vi "Day05-1.vi"() -> ()   [LabVIEW 2021]
panel:
  out "points with at least two lines overlap":i32
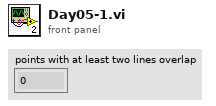
[diagram p1: front panel]
types:
  T1 = cluster{"[0]":i32, "[1]":i32, "[2]":i32, "[3]":i32, "[4]":i32, "[5]":i32, "[6]":i32, "[7]":i32, "[8]":i32}
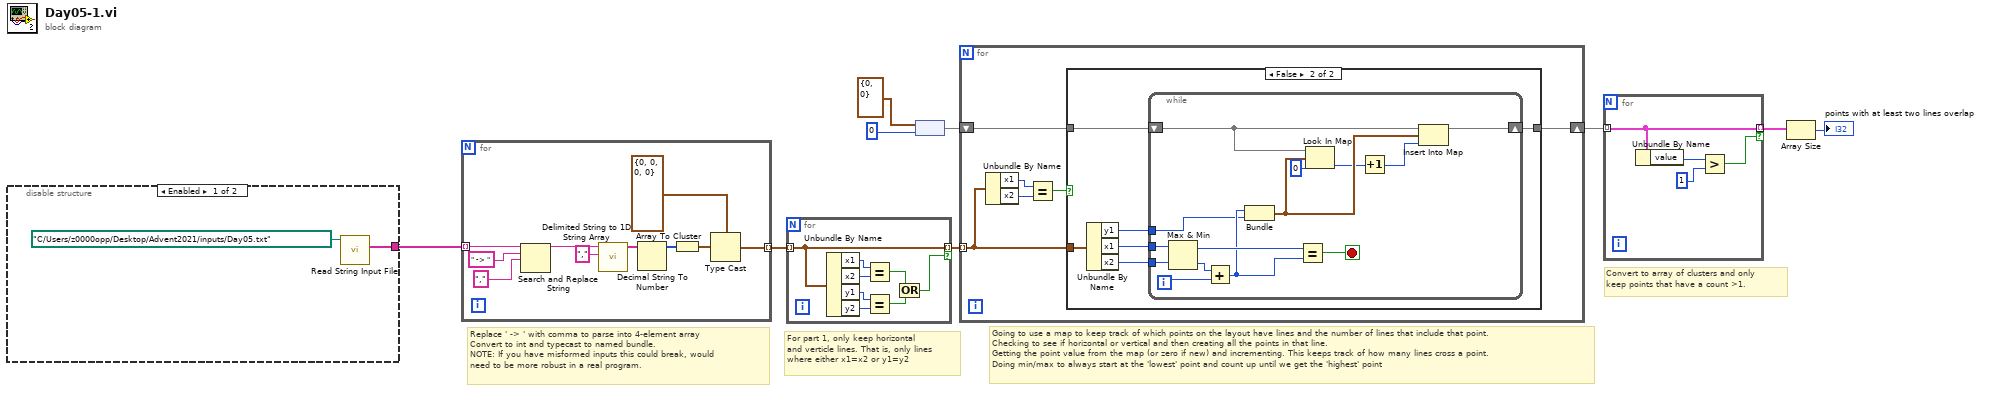
[diagram p0: block diagram]
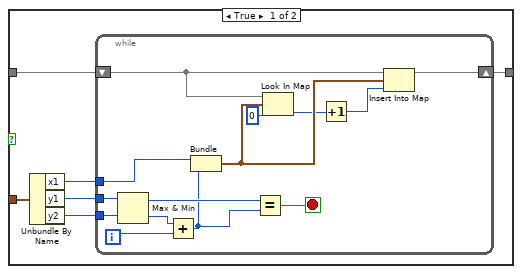
[diagram p2: hidden frame]
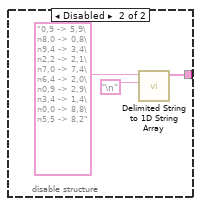
[diagram p3: hidden frame]
diagram:
  # "Convert to array of clusters and only\nkeep points that have a count >1."
  # "Going to use a map to keep track of which points on the layout have lines and the number of lines that include that point.\nChecking to see if horizontal or vertical and then creating all the points in that line.\nGetting the point value from the map (or zero if new) and incrementing. This keeps track of how many lines cross a point.\nDoing min/max to always start at the 'lowest' point and count up until we get the 'highest' point"
  # "For part 1, only keep horizontal\nand verticle lines. That is, only lines\nwhere either x1=x2 or y1=y2"
  # "Replace ' -> ' with comma to parse into 4-element array\nConvert to int and typecast to named bundle.\nNOTE: If you have misformed inputs this could break, would\nneed to be more robust in a real program."
  n1 = disable-structure shown="Enabled" {
    disable-tunnel: [w10 w12] -> w9
    frame Enabled {
      n2 = call "Read String Input File.vi"("file path (dialog if empty)"=path "C:/Users/z0000opp/Desktop/Advent2021/inputs/Day05.txt") -> ("input values"=w10:string[])  [unwired: 10 in]
    }
    frame Disabled {
      n3 = call <vilib>:"Delimited String to 1D String Array.vi"("delimiter"="\n", "delimited string"="0,9 -> 5,9\n8,0 -> 0,8\n9,4 -> 3,4\n2,2 -> 2,1\n7,0 -> 7,4\n6,4 -> 2,0\n0,9 -> 2,9\n3,4 -> 1,4\n0,0 -> 8,8\n5,5 -> 8,2") -> ("string array"=w12:string[])  [unwired: 9 in]
    }
  }
  n4 = for {
    tunnel: w9 -> [w24] mode=indexing
    tunnel: [w15] -> w8 mode=indexing
    n5 = Search and Replace String(input string=w24, search string=" -> ", replace string=",") -> (result string=w21:string)  [unwired: 5 in, 3 out]
    n6 = call <vilib>:"Delimited String to 1D String Array.vi"("delimiter"=",", "delimited string"=w21) -> ("string array"=w19:string[])  [unwired: 9 in]
    n7 = Decimal String To Number(string=w19) -> (number=w18:i32[])  [unwired: 2 in, 1 out]
    n8 = Array To Cluster(array=w18) -> (cluster=w17:T1)
    n9 = Type Cast(type=cluster{"x1":i32, "y1":i32, "x2":i32, "y2":i32} {"x1"=0, "y1"=0, "x2"=0, "y2"=0}, x=w17) -> (*(type *) &x=w15:cluster{"x1":i32, "y1":i32, "x2":i32, "y2":i32})
  }
  n10 = for {
    tunnel: w8 -> [w26] mode=indexing
    tunnel: [w26] -> w7 mode=indexing if=w25
    n11 = Unbundle By Name(w26) -> ("x1"=w31:i32, "x2"=w32:i32, "y1"=w30:i32, "y2"=w29:i32)
    n12 = Equal?(x=w31, y=w32) -> (x = y?=w27:bool)
    n13 = Equal?(x=w30, y=w29) -> (x = y?=w28:bool)
    n14 = Or(x=w27, y=w28) -> (x .or. y?=w25:bool)
  }
  n15 = node(cluster{"x":i32, "y":i32} {"x"=0, "y"=0}, 0) -> (w6:map{cluster{"x":i32, "y":i32}, i32})
  n16 = for {
    tunnel: w7 -> [w35] mode=indexing
    shift-right: [w33] -> w3
    shift-left: w6 -> [w34]
    n17 = Unbundle By Name(w35) -> ("x1"=w37:i32, "x2"=w38:i32)
    n18 = Equal?(x=w37, y=w38) -> (x = y?=w36:bool)
    n19 = case shown="False" w36 {
      tunnel: w35 -> [w44 w64]
      tunnel: w34 -> [w43 w63]
      tunnel: [w39 w59] -> w33
      frame True {
        n20 = Unbundle By Name(w44) -> ("x1"=w42:i32, "y1"=w41:i32, "y2"=w40:i32)
        n21 = while {
          shift-right: [w48] -> w39
          shift-left: w43 -> [w52]
          tunnel: w42 -> [w56]
          tunnel: w41 -> [w58]
          tunnel: w40 -> [w57]
          i -> [w54]
          stop <- w45 stop-if-true
          n22 = Max & Min(x=w58, y=w57) -> (max(x,y)=w47:i32, min(x,y)=w55:i32)
          n23 = Add(x=w55, y=w54) -> (x+y=w46:i32)
          n24 = Bundle("x1"=w56, w46) -> (w51:cluster{"x1":i32, i32})  [unwired: 1 in]
          n25 = Equal?(x=w47, y=w46) -> (x = y?=w45:bool)
          n26 = Look In Map(map=w52, key=w51, default value=0) -> (value=w50:i32)  [unwired: 1 out]
          n27 = Increment(x=w50) -> (x+1=w49:i32)
          n28 = Insert Into Map(map in=w52, key=w51, value=w49) -> (map out=w48:map{cluster{"x":i32, "y":i32}, i32})  [unwired: 2 out]
        }
      }
      frame False {
        n29 = Unbundle By Name(w64) -> ("y1"=w62:i32, "x1"=w61:i32, "x2"=w60:i32)
        n30 = while {
          shift-right: [w69] -> w59
          shift-left: w63 -> [w73]
          tunnel: w62 -> [w65]
          tunnel: w61 -> [w78]
          tunnel: w60 -> [w77]
          i -> [w75]
          stop <- w67 stop-if-true
          n31 = Max & Min(x=w78, y=w77) -> (max(x,y)=w68:i32, min(x,y)=w76:i32)
          n32 = Add(x=w76, y=w75) -> (x+y=w66:i32)
          n33 = Bundle(w66, "y1"=w65) -> (w72:cluster{i32, "y1":i32})  [unwired: 1 in]
          n34 = Equal?(x=w68, y=w66) -> (x = y?=w67:bool)
          n35 = Look In Map(map=w73, key=w72, default value=0) -> (value=w71:i32)  [unwired: 1 out]
          n36 = Increment(x=w71) -> (x+1=w70:i32)
          n37 = Insert Into Map(map in=w73, key=w72, value=w70) -> (map out=w69:map{cluster{"x":i32, "y":i32}, i32})  [unwired: 2 out]
        }
      }
    }
  }
  n38 = for {
    tunnel: [w82] -> w2 mode=indexing if=w79
    tunnel: w3 -> [w82] mode=indexing
    n39 = Unbundle By Name(w82) -> ("value"=w81:i32)
    n40 = Greater?(x=w81, y=1) -> (0:w79:bool)
  }
  n41 = Array Size(array=w2) -> (size(s)=→"points with at least two lines overlap":i32)
